vi "LogForDuration.vi"(6 "Rate [Hz]":dbl=100.0, 7 "Log File Path (temporary file)":path, 8 "error in (no error)":errorcluster, 9 "milliseconds to wait":u32=1000, 10 "Channel Paths":string[](array[string]), 11 "WorkspaceManager":T1) -> (0 "error out":errorcluster, 2 "data":waveform(dbl)[](array[waveform]), 3 "WorkspaceManager out":T1)   [LabVIEW 2015, in "VeriStandTestUtilities.lvlib"]
uses:
  VeriStandTestUtilities.lvlib
  <vilib>/NI Veristand/Execution/Workspace/WorkspaceAPI.ctl
  NationalInstruments.VeriStand.ClientAPI
  <vilib>/NI VeriStand/Execution/Workspace/NI_VS Workspace ExecutionAPI.lvlib
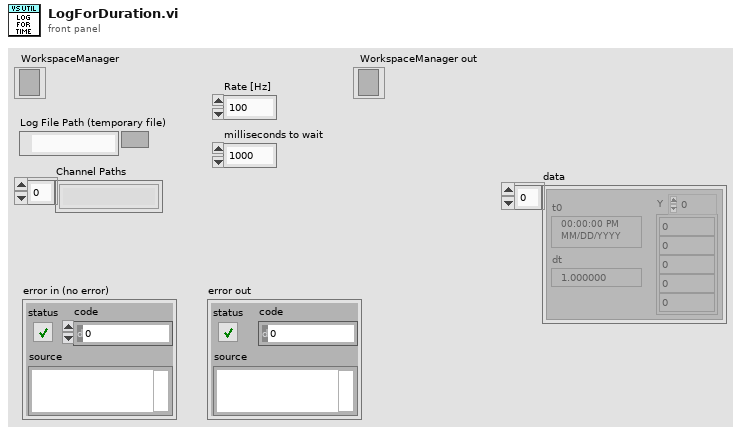
[diagram p1: front panel]
types:
  T1 = typedef "NI_VS Workspace ExecutionAPI.lvlib/WorkspaceAPI.ctl" = refnum<k24>
  T2 = typedef "NI_VS Workspace ExecutionAPI.lvlib/LogFileConfiguration.ctl" = cluster{"File Path":path, "Description":string, "Trigger":T3, "Replace File":bool, "Rate [Hz]":dbl, "File Properties":T5[], "Channels":T6[]}
  T3 = typedef "NI_VS Workspace ExecutionAPI.lvlib/LogFileTriggerConfiguration.ctl" = cluster{"Type":T4, "Channel Path":string, "High Limit":dbl, "Low Limit":dbl}
  T4 = typedef "NI_VS Workspace ExecutionAPI.lvlib/LogFileTriggerType.ctl" = enum16{"None", "In Limits", "Out of Limits"}
  T5 = typedef "NI_VS Workspace ExecutionAPI.lvlib/LogProperty.ctl" = cluster{"Name":string, "Value":string}
  T6 = typedef "NI_VS Workspace ExecutionAPI.lvlib/LogChannelConfiguration.ctl" = cluster{"Channel Path":string, "Custom Name":string, "Custom Group":string, "Properties":T5[]}
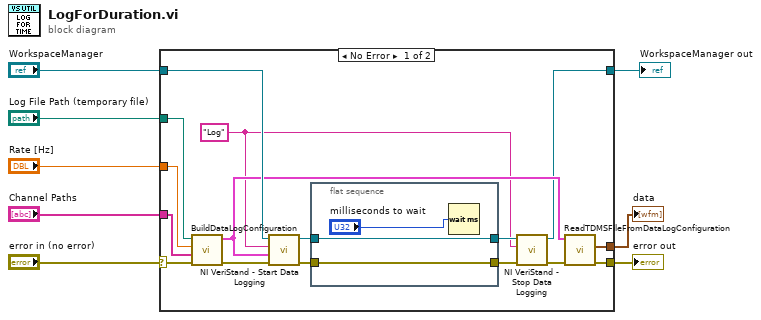
[diagram p0: block diagram]
diagram:
  n1 = case shown="No Error" "error in (no error)" {
    selector: "error in (no error)" -> [w15 w29]
    tunnel: [w24 w29] -> w8
    tunnel: [w11 w28] -> w1
    tunnel: [w23 _] -> w7
    tunnel: "Channel Paths" -> [w22 _]
    tunnel: "Log File Path (temporary file)" -> [w19 _]
    tunnel: "Rate [Hz]" -> [w18 _]
    tunnel: "WorkspaceManager" -> [w16 w28]
    frame No Error {
      w9 = "Log" ("Data Log Configuration Name")
      n2 = call "BuildDataLogConfiguration.vi"("error in (no error)"=w15, "Channel Paths"=w22, "Rate [Hz]"=w18, "Log File Path (temporary file)"=w19) -> ("error out"=w17:errorcluster, "Data Log File Configuration"=w14:T2)  [unwired: 6 in]
      n3 = call <vilib>:"NI VeriStand - Start Data Logging.vi"("error in (no error)"=w17, "Data Log File Configuration"=w14, "Data Log Configuration Name"=w9, "WorkspaceManager in"=w16) -> ("error out"=w20:errorcluster, "WorkspaceManager out"=w21:T1)  [unwired: 6 in]
      n4 = flat-sequence {
        tunnel: w20 -> [w27]
        tunnel: [w27] -> w13
        tunnel: w21 -> [w26]
        tunnel: [w26] -> w10
        frame #0 {
          n5 = Wait (ms)(milliseconds to wait="milliseconds to wait") -> ()  [unwired: 1 out]
        }
      }
      n6 = call <vilib>:"NI VeriStand - Stop Data Logging.vi"("error in (no error)"=w13, "Data Log Configuration Name"=w9, "WorkspaceManager in"=w10) -> ("error out"=w12:errorcluster, "WorkspaceManager out"=w11:T1)  [unwired: 7 in]
      n7 = call "ReadTDMSFileFromDataLogConfiguration.vi"("error in (no error)"=w12, "Data Log File Configuration"=w14) -> ("error out"=w24:errorcluster, "data"=w23:waveform(dbl)[])  [unwired: 7 in, 1 out]
    }
    frame Error {
    }
  }
  "error out" <- w8
  "data" <- w7
  "WorkspaceManager out" <- w1
